vi "FC to XY.vi"(6 "scaling":dbl=1.37 format="%#_13g", 9 "all rows":dbl[][](array[numeric]), 10 "Numeric":dbl, 11 "Numeric 2":dbl) -> (3 "Array":cluster{dbl[], dbl[]}[](array[cluster]))   [LabVIEW 2015]
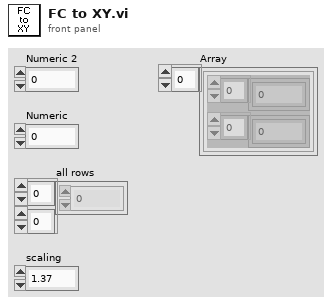
[diagram p1: front panel]
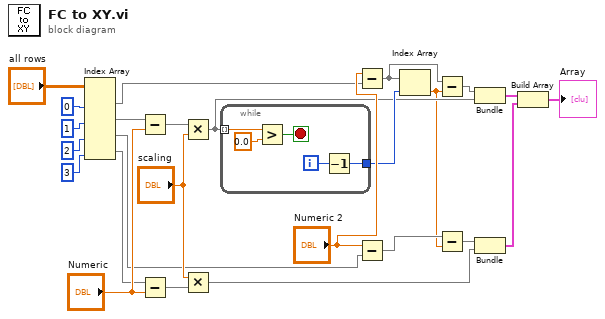
[diagram p0: block diagram]
diagram:
  n1 = Index Array(array="all rows", index (col) #1=0 ("disabled index (col)"), index (col) #2=1 ("index (col)"), index (col) #3=2 ("index (col)"), index (col) #4=3 ("index (col)")) -> (element #1=w14:dbl[], element #2=w17:dbl[], element #3=w15:dbl[], element #4=w18:dbl[])  [unwired: 4 in]
  n2 = Subtract(x=w17, y="Numeric") -> (x-y=w24:dbl[])
  n3 = Subtract(x=w18, y="Numeric") -> (x-y=w22:dbl[])
  n4 = Multiply(x=w24, y="scaling") -> (x*y=w6:dbl[])
  n5 = Multiply(x="scaling", y=w22) -> (x*y=w23:dbl[])
  n6 = while {
    tunnel: w6 -> [w30] mode=indexing
    tunnel: [w27] -> w7
    i -> [w26]
    stop <- w28 stop-if-true
    n7 = Greater?(x=w30, y=0.0) -> (0:w28:bool)
    n8 = Decrement(x=w26) -> (x-1=w27:i32)
  }
  n9 = Subtract(x="Numeric 2", y=w14) -> (x-y=w8:dbl[])
  n10 = Subtract(x="Numeric 2", y=w15) -> (x-y=w3:dbl[])
  n11 = Index Array(array=w8, index=w7) -> (element=w1:dbl)
  n12 = Subtract(x=w8, y=w1) -> (x-y=w5:dbl[])
  n13 = Subtract(x=w3, y=w1) -> (x-y=w2:dbl[])
  n14 = Bundle(w5, w6) -> (w9:cluster{dbl[], dbl[]})  [unwired: 1 in]
  n15 = Bundle(w2, w23) -> (w4:cluster{dbl[], dbl[]})  [unwired: 1 in]
  n16 = Build Array(w9, w4) -> (→"Array":cluster{dbl[], dbl[]}[])
